vi "Hold and Measure_Save Sweep Data to csv.vi"(5 "Selected Exp Settings":T5={"Floor_Sweep_Stop_V"=36.0, "Resistance Threshold"=1.0, "Floor_Sweep_Start_V"=36.0, "Floor_Sweep_Step_V"=1.0, "Roof_Sweep_Stop_V"=36.0, "Roof_Sweep_Start_V"=36.0, "Roof_Sweep_Step_V"=1.0, "Experiment Name"="", "Meas_Type"=[0, 2, 4]}, 6 "Additional Data":T7, 7 "Filepath":path, 8 "Time":dbl[](array[numeric]), 9 "Data Management Control":T3, 10 "Date Cluster":T4, 11 "Test Information":T2={"Exp Name"="Cold Switching", "Lot"="0233A", "Wafer"="15", "Die Type"="L22", "Die X "="6", "Die Y"="8", "Exp"="1", "Die X_Y"="8"}) -> ()   [LabVIEW 2013]
uses:
  Controls/Date Control.ctl
  Controls/Data Management.ctl
  Controls/Test Information.ctl
  Controls/Additional Data.ctl
  Controls/Individual User Inputs_MultiTest.ctl
  Controls/Test Selection.ctl
  <vilib>/Utility/file.llb/Write To Spreadsheet File (string).vi
panel:
  in  "Tab Control":T1(tab)
  # "Calculation Settings"
  # "Test Settings"
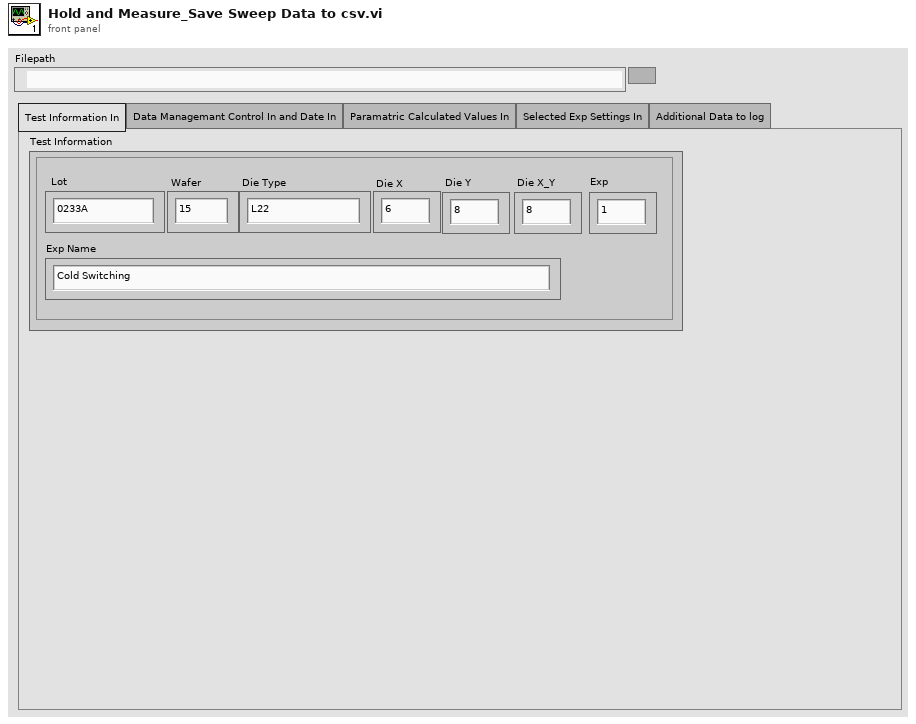
[diagram p1: front panel]
types:
  T1 = enum32{"Test Information In", "Data Managemant Control In and Date In", "Paramatric Calculated Values In", "Selected Exp Settings In", "Additional Data to log"}
  T2 = typedef "Test Information.ctl" = cluster{"Exp Name":string, "Lot":string, "Wafer":string, "Die Type":string, "Die X ":string, "Die Y":string, "Exp":string, "Die X_Y":string}
  T3 = typedef "Data Management.ctl" = cluster{"Bias_Voltage Sweep":dbl[], "CPD":dbl[], "DMM_Measurement_V":dbl[], "Port 1 Capacitance":dbl[], "Port 2 Capacitance":dbl[], "Bias_Voltage Measurement":dbl[], "Bias_Current Measurement":dbl[], "Contact_Source_Current":dbl[], "Contact_Sink_Current":dbl[], "Calculated Resitance":dbl[]}
  T4 = typedef "Date Control.ctl" = cluster{"Date":string, "Start Time":string, "Stop Time":string}
  T5 = typedef "Individual User Inputs_MultiTest.ctl" = cluster{"Floor_Sweep_Stop_V":dbl, "Resistance Threshold":dbl, "Floor_Sweep_Start_V":dbl, "Floor_Sweep_Step_V":dbl, "Roof_Sweep_Stop_V":dbl, "Roof_Sweep_Start_V":dbl, "Roof_Sweep_Step_V":dbl, "Experiment Name":string, "Meas_Type":T6}
  T6 = typedef "Test Selection.ctl" = i32[]
  T7 = typedef "Additional Data.ctl" = cluster{"P2_Capacitance_PostTest":dbl[], "P1_Capacitance _PostTest":dbl[], "P1_Capacitance_PreTest":dbl[], "P2_Capacitance_PreTest":dbl[]}
  T8 = enum16{"open", "replace", "create", "open or create", "replace or create", "replace or create with confirmation"}
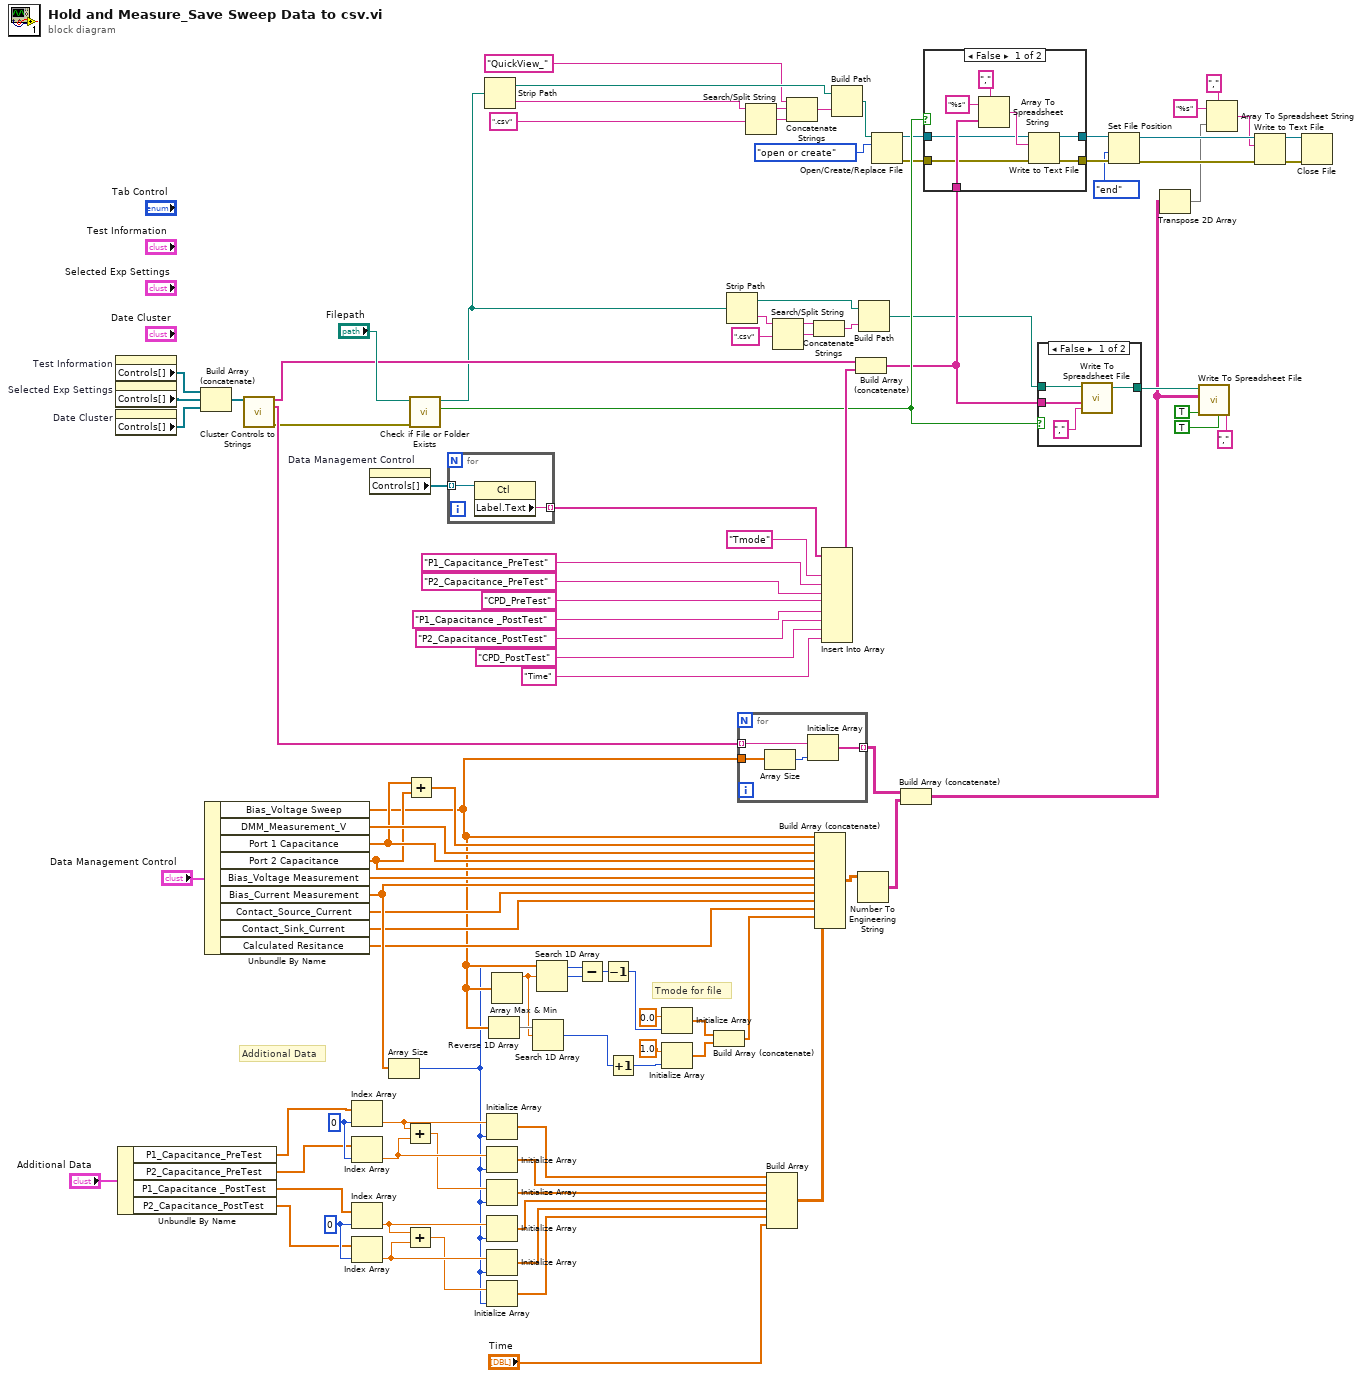
[diagram p0: block diagram]
diagram:
  w48 = 0 ("index")
  w49 = 0 ("index")
  # "Additional Data"
  # "Tmode for file"
  n1 = property on="Test Information" class="Clust (strict)"() -> ("Controls[]"=w104:refnum<vi>[])  [unwired: 2 in, 2 out]
  n2 = property on="Selected Exp Settings" class="Clust (strict)"() -> ("Controls[]"=w1:refnum<vi>[])  [unwired: 2 in, 2 out]
  n3 = property on="Date Cluster" class="Clust (strict)"() -> ("Controls[]"=w102:refnum<vi>[])  [unwired: 2 in, 2 out]
  n4 = Unbundle By Name("Additional Data") -> ("P1_Capacitance_PreTest"=w27:dbl[], "P2_Capacitance_PreTest"=w26:dbl[], "P1_Capacitance _PostTest"=w25:dbl[], "P2_Capacitance_PostTest"=w24:dbl[])
  n5 = Build Array (concatenate)(w104, w1, w102) -> (w103:refnum<vi>[])
  n6 = Unbundle By Name("Data Management Control") -> ("Bias_Voltage Sweep"=w12:dbl[], "DMM_Measurement_V"=w98:dbl[], "Port 1 Capacitance"=w15:dbl[], "Port 2 Capacitance"=w14:dbl[], "Bias_Voltage Measurement"=w97:dbl[], "Bias_Current Measurement"=w96:dbl[], "Contact_Source_Current"=w53:dbl[], "Contact_Sink_Current"=w52:dbl[], "Calculated Resitance"=w50:dbl[])
  n7 = call "Cluster Controls to Strings.vi"("Controls[]"=w103) -> ("Control Labels"=w80:string[], "Control Values"=w100:string[], "Error Out"=w79:errorcluster)  [unwired: 12 in]
  n8 = Index Array(array=w27, index=w49) -> (element=w47:dbl)
  n9 = Index Array(array=w26, index=w49) -> (element=w46:dbl)
  n10 = Index Array(array=w25, index=w48) -> (element=w44:dbl)
  n11 = Index Array(array=w24, index=w48) -> (element=w43:dbl)
  n12 = property on="Data Management Control" class="Clust (strict)"() -> ("Controls[]"=w92:refnum<vi>[])  [unwired: 2 in, 2 out]
  n13 = Array Size(array=w96) -> (size(s)=w7:i32)
  n14 = Add(x=w47, y=w46) -> (x+y=w45:dbl)
  n15 = Add(x=w44, y=w43) -> (x+y=w42:dbl)
  n16 = Add(x=w15, y=w14) -> (x+y=w13:dbl[])
  n17 = call <vilib>:"Check if File or Folder Exists.vi"("error in (no error)"=w79, "path"="Filepath") -> ("file or folder exists?"=w69:bool, "dup path"=w17:path)  [unwired: 7 in, 1 out]
  n18 = for {
    tunnel: w92 -> [w106] mode=indexing
    tunnel: [w105] -> w85 mode=indexing
    n19 = property class="Ctl"(reference=w106) -> ("Label.Text"=w105:string)  [unwired: 1 in, 2 out]
  }
  n20 = Strip Path(path=w17) -> (stripped path=w74:path, name=w77:string)
  n21 = Initialize Array(w47, w7) -> (w41:dbl[])
  n22 = Initialize Array(w46, w7) -> (w40:dbl[])
  n23 = Initialize Array(w45, w7) -> (w39:dbl[])
  n24 = Initialize Array(w44, w7) -> (w38:dbl[])
  n25 = Initialize Array(w43, w7) -> (w37:dbl[])
  n26 = Initialize Array(w42, w7) -> (w36:dbl[])
  n27 = Reverse 1D Array(array=w12) -> (reversed array=w11:dbl[])
  n28 = Array Max & Min(array=w12) -> (max value=w10:dbl)  [unwired: 3 out]
  n29 = Search 1D Array(1D array=w11, element=w10) -> (index of element=w3:i32)  [unwired: 1 in]
  n30 = Search 1D Array(1D array=w12, element=w10) -> (index of element=w6:i32)  [unwired: 1 in]
  n31 = Subtract(x=w7, y=w6) -> (x-y=w5:i32)
  n32 = Decrement(x=w5) -> (x-1=w4:i32)
  n33 = Increment(x=w3) -> (x+1=w2:i32)
  n34 = Initialize Array(0.0, w4) -> (w99:dbl[])
  n35 = Initialize Array(1.0, w2) -> (w93:dbl[])
  n36 = Build Array (concatenate)(w99, w93) -> (w51:dbl[])
  n37 = Strip Path(path=w17) -> (stripped path=w20:path, name=w23:string)
  n38 = for {
    tunnel: w12 -> [w110]
    tunnel: w100 -> [w109] mode=indexing
    tunnel: [w107] -> w87 mode=indexing
    n39 = Array Size(array=w110) -> (size(s)=w108:i32)
    n40 = Initialize Array(w109, w108) -> (w107:string[])
  }
  n41 = Search/Split String(string=w77, search string/char (-)=".csv" ("search string")) -> (substring before match=w72:string, match + rest of string=w75:string)  [unwired: 1 in, 1 out]
  n42 = Build Array(w41, w40, w39, w38, w37, w36, "Time") -> (w35:dbl[][])
  n43 = Search/Split String(string=w23, search string/char (-)=".csv" ("search string")) -> (substring before match=w18:string, match + rest of string=w21:string)  [unwired: 1 in, 1 out]
  n44 = Concatenate Strings("QuickView_" ("search string"), w72, w75) -> (w73:string)
  n45 = Concatenate Strings(w18, w21) -> (w19:string)
  n46 = Build Array (concatenate)(w12, w13, w98, w15, w14, w97, w96, w53, w52, w50, w51, w35) -> (w82:dbl[][])
  n47 = Insert Into Array(array=w85, new element #1="Tmode" ("new element/subarray"), new element #2="P1_Capacitance_PreTest" ("new element/subarray"), new element #3="P2_Capacitance_PreTest" ("new element/subarray"), new element #4="CPD_PreTest" ("new element/subarray"), new element #5="P1_Capacitance _PostTest" ("new element/subarray"), new element #6="P2_Capacitance_PostTest" ("new element/subarray"), new element #7="CPD_PostTest" ("new element/subarray"), new element #8="Time" ("new element/subarray")) -> (w84:string[])  [unwired: 1 in]
  n48 = Build Path(base path=w74, name or relative path=w73) -> (appended path=w70:path)
  n49 = Build Array (concatenate)(w80, w84) -> (w68:string[])
  n50 = Number To Engineering String(4:w82) -> (0:w86:string[][])  [unwired: 3 in]
  n51 = Build Path(base path=w20, name or relative path=w19) -> (appended path=w16:path)
  n52 = Open/Create/Replace File(file path (use dialog)=w70, operation (0:open)=T8."open or create") -> (refnum out=w67:refnum<file>, error out=w66:errorcluster)  [unwired: 4 in, 1 out]
  n53 = Build Array (concatenate)(w87, w86) -> (w55:string[][])
  n54 = case shown="False" w69 {
    tunnel: w68 -> [w116 _]
    tunnel: w67 -> [w114 w120]
    tunnel: w66 -> [w113 w119]
    tunnel: [w112 w119] -> w64
    tunnel: [w111 w120] -> w65
    frame False {
      n55 = Array To Spreadsheet String(delimiter (Tab)="," ("delimiter (\\t)"), array=w116, 3:"%s" ("format string")) -> (spreadsheet string=w115:string)
      n56 = Write to Text File(file (use dialog)=w114, text=w115, error in=w113) -> (refnum out=w111:refnum<file>, error out=w112:errorcluster)  [unwired: 1 in, 1 out]
    }
    frame True {
    }
  }
  n57 = case shown="False" w69 {
    tunnel: w16 -> [w124 w125]
    tunnel: w68 -> [w123 _]
    tunnel: [w121 w125] -> w91
    frame False {
      n58 = call-poly <vilib>:"Write To Spreadsheet File.vi"("delimiter (\\t)"="," ("delimiter (\\t)"), "1D data"=w123, "file path (dialog if empty)"=w124) -> ("new file path (Not A Path if cancelled)"=w121:path)  [unwired: 5 in]
    }
    frame True {
    }
  }
  n59 = Set File Position(refnum=w65, from (0:start)=enum16{"start", "end", "current"}."end", error in=w64) -> (refnum out=w59:refnum<file>, error out=w60:errorcluster)  [unwired: 1 in]
  n60 = Transpose 2D Array(2D array=w55) -> (transposed array=w54:string[][])
  n61 = call-poly <vilib>:"Write To Spreadsheet File.vi"("delimiter (\\t)"="," ("delimiter (\\t)"), "transpose? (no:F)"=TRUE, "append to file? (new file:F)"=TRUE, "2D data"=w55, "file path (dialog if empty)"=w91) -> ()  [unwired: 3 in, 1 out]
  n62 = Array To Spreadsheet String(delimiter (Tab)="," ("delimiter (\\t)"), array=w54, 3:"%s" ("format string")) -> (spreadsheet string=w58:string)
  n63 = Write to Text File(file (use dialog)=w59, text=w58, error in=w60) -> (refnum out=w56:refnum<file>, error out=w57:errorcluster)  [unwired: 1 in, 1 out]
  n64 = Close File(refnum=w56, error in=w57) -> ()  [unwired: 2 out]
